vi "MySubsystem_Global.vi"() -> ()   [LabVIEW 2020]
panel:
  in  "Cals/MySubsystem/StringVariable1":string
  in  "Cals/MySubsystem/BoolVariable1":bool
  in  "Cals/MySubsystem/DblVariable3":dbl
  in  "Cals/MySubsystem/DblVariable2":dbl
  in  "Cals/MySubsystem/DblVariable1":dbl
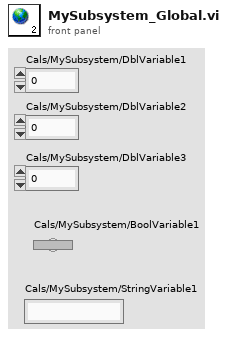
[diagram p1: front panel]
diagram:
